vi "Result_Test.vi"(8 "error in (no error)":errorcluster caption="entrée d'erreur (pas d'erreur)", 11 "Get_Voltage en entrée":refnum<class "P2056_Set_SN_PCBA.lvclass">) -> (0 "error out":errorcluster caption="sortie d'erreur", 3 "Get_Voltage en sortie":refnum<class "P2056_Set_SN_PCBA.lvclass">)   [LabVIEW 2020, in "Library Test.lvlib" / "P2056_Set_SN_PCBA.lvclass"]
uses:
  P2056_Set_SN_PCBA.lvclass
  C:/Users/ngarcin/OneDrive - Altyor/Standard TB/Class/Test/Test (Default)/Test (Default).lvclass
  JSON API/JSON Value/Set from JSON string.vi
  JSON API/JSON Value/JSON Value.lvclass
  P2056_Send_Command_UART.lvclass
  P2056_Set_SN_PCBA.lvclass/P2056_Set_SN_PCBA.ctl
  JSON API/Variant JSON/Variant JSON.lvlib
  JSON API/Get Polymorphic/JSON GetSet.lvlib
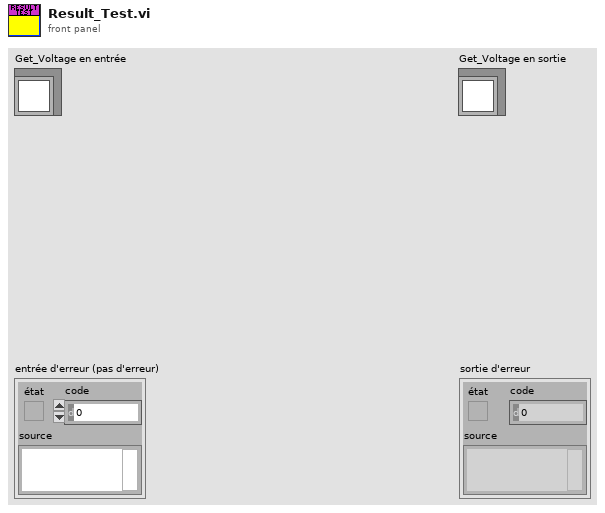
[diagram p1: front panel]
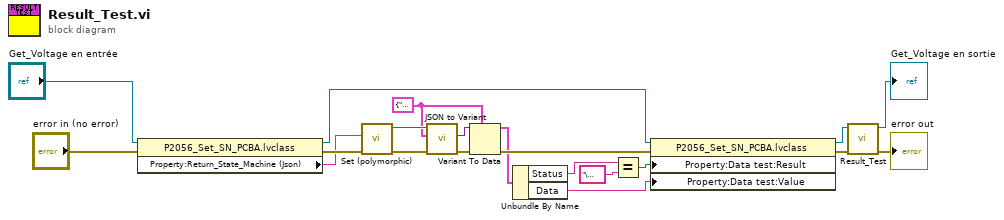
[diagram p0: block diagram]
diagram:
  w14 = cluster{"Data":string, "Status":string} {"Data"="", "Status"=""}
  n1 = property class="P2056_Set_SN_PCBA.lvclass"(reference="Get_Voltage en entrée", error in="error in (no error)") -> (reference out=w19:refnum<class "P2056_Set_SN_PCBA.lvclass">, error out=w13:errorcluster, "Property:Return_State_Machine (Json)"=w11:string)
  n2 = call-poly "Set (polymorphic).vi"("error in (no error)"=w13, "JSON stream"=w11) -> ("error out"=w16:errorcluster, "JSON Value out"=w18:refnum<class "JSON Value.lvclass">)  [unwired: 7 in, 1 out]
  n3 = call "JSON to Variant.vi"("error in (no error)"=w16, "Variant (Data Type)"=w14, "JSON Value"=w18) -> ("error out"=w17:errorcluster, "Variant out"=w15:variant)  [unwired: 7 in]
  n4 = Variant To Data(error in=w17, type=w14, Variant=w15) -> (data=w10:cluster{"Data":string, "Status":string}, error out=w12:errorcluster)
  n5 = Unbundle By Name(w10) -> ("Status"=w9:string, "Data"=w6:string)
  n6 = Equal?(x=w9, y="\u0000") -> (x = y?=w7:bool)
  n7 = property class="P2056_Set_SN_PCBA.lvclass"(reference=w19, error in=w12, "Property:Data test:Result"=w7, "Property:Data test:Value"=w6) -> (reference out=w4:refnum<class "P2056_Set_SN_PCBA.lvclass">, error out=w5:errorcluster)
  n8 = call-parent "Result_Test.vi"("error in (no error)"=w5, "Get_Voltage en entrée"=w4) -> ("error out"=→"error out":errorcluster, "Get_Voltage en sortie"=→"Get_Voltage en sortie":refnum<class "P2056_Set_SN_PCBA.lvclass">)  [unwired: 8 in]
